vi "Select Colors.vi"(9 "Color Select":T2, 11 "State":T3) -> (1 "Text Colors":T1, 3 "Button Colors":cluster{"FG":u32, "BG":u32}[](array[cluster]))   [LabVIEW 2012, in "Hover Button.xctl"]
doc: "This vi is used to convert a color set from the State data to a format that can be written to the Boolean button element of the Hover Button."
uses:
  Hover Button.xctl
  State.ctl
  Button Colors.ctl
  Font Properties.ctl
  Color Select.ctl
panel:
  # "This vi selects the color set in the color\nrelated State data to convert to the\nformat required for the Boolean button\nproperties"
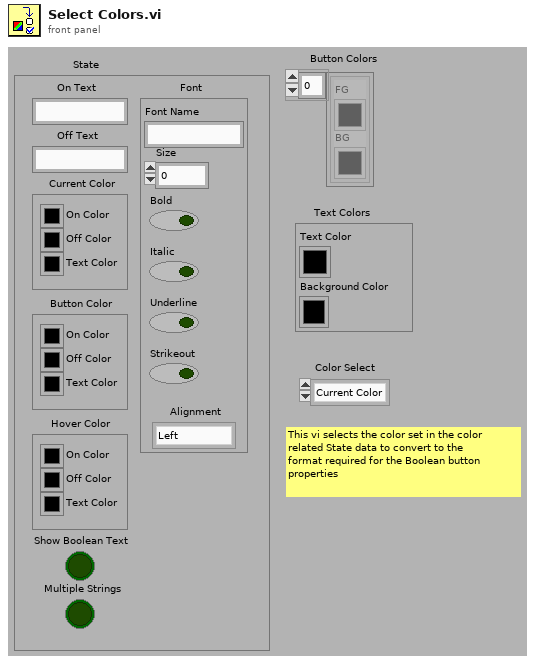
[diagram p1: front panel]
types:
  T1 = cluster{"Text Color":u32, "Background Color":u32}
  T2 = typedef "Hover Button.xctl/Color Select.ctl" = enum16{"Current Color", "Button Color", "Hover Color"}
  T3 = typedef "Hover Button.xctl/State.ctl" = cluster{"On Text":string, "Off Text":string, "Current Color":T4, "Button Color":T4, "Hover Color":T4, "Show Boolean Text":bool, "Multiple Strings":bool, "Font":T5}
  T4 = typedef "Hover Button.xctl/Button Colors.ctl" = cluster{"On Color":u32, "Text Color":u32, "Off Color":u32}
  T5 = typedef "Hover Button.xctl/Font Properties.ctl" = cluster{"Font Name":string, "Size":u32, "Bold":bool, "Italic":bool, "Underline":bool, "Strikeout":bool, "Alignment":enum16{"Left", "Center", "Right"}}
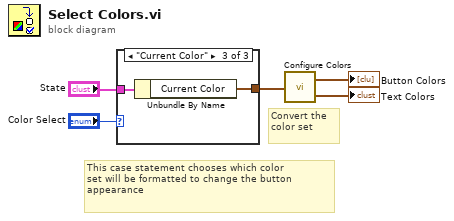
[diagram p0: block diagram]
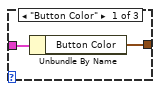
[diagram p2: hidden frame]
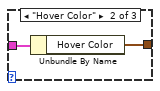
[diagram p3: hidden frame]
diagram:
  # "Convert the\ncolor set"
  # "This case statement chooses which color\nset will be formatted to change the button\nappearance"
  n1 = case shown="\"Current Color\"" "Color Select" {
    tunnel: "State" -> [w7 w9 w11]
    tunnel: [w6 w8 w10] -> w3
    frame "Button Color" {
      n2 = Unbundle By Name(w7) -> ("Button Color"=w6:T4)
    }
    frame "Hover Color" {
      n3 = Unbundle By Name(w9) -> ("Hover Color"=w8:T4)
    }
    frame "Current Color" {
      n4 = Unbundle By Name(w11) -> ("Current Color"=w10:T4)
    }
  }
  n5 = call "Configure Colors.vi"("Current Color"=w3) -> ("Array"=→"Button Colors":cluster{"FG":u32, "BG":u32}[], "Text Colors"=→"Text Colors":T1)
